vi "etlReadOpen.vi"   [LabVIEW 2017]
uses:
  globalDevices.vi
  <vilib>/DAQmx/create/channels.llb/DAQmx Create Channel (AI-Voltage-Basic).vi
  <vilib>/DAQmx/configure/timing.llb/DAQmx Timing (Sample Clock).vi
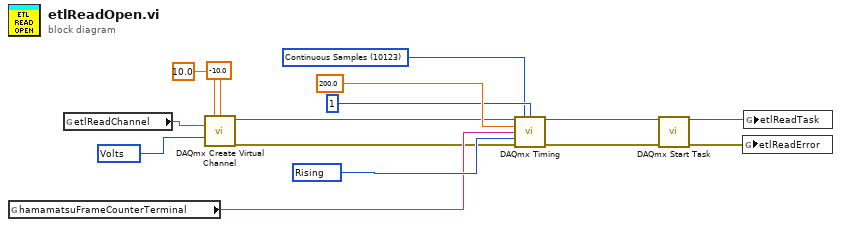
[diagram p0: block diagram]
diagram:
  w10 = 10348 items=["Volts"=10348, "From Custom Scale"=10065] ("units")
  w15 = 10280 items=["Rising"=10280, "Falling"=10171] ("active edge")
  w11 = 10123 items=["Finite Samples"=10178, "Continuous Samples"=10123, "Hardware Timed Single Point"=12522] ("sample mode")
  n1 = global read "globalDevices.vi" "hamamatsuFrameCounterTerminal"() -> (w14:tag)
  n2 = global read "globalDevices.vi" "etlReadChannel"() -> (w1:tag)
  n3 = call-poly <vilib>:"DAQmx Create Virtual Channel.vi"("maximum value"=10.0, "minimum value"=-10.0, "physical channels"=w1, "units"=w10) -> ("task out"=w6:refnum<k21>, "error out"=w7:errorcluster)  [unwired: 10 in]
  n4 = call-poly <vilib>:"DAQmx Timing.vi"("task/channels in"=w6, "sample mode"=w11, "samples per channel"=1, "rate"=200.0, "source"=w14, "active edge"=w15, "error in"=w7) -> ("task out"=w8:refnum<k21>, "error out"=w9:errorcluster)  [unwired: 7 in]
  n5 = call <vilib>:"DAQmx Start Task.vi"("task/channels in"=w8, "error in"=w9) -> ("task out"=w3:refnum<k21>, "error out"=w2:errorcluster)  [unwired: 12 in]
  n6 = global write "globalDevices.vi" "etlReadError"(w2) -> ()
  n7 = global write "globalDevices.vi" "etlReadTask"(w3) -> ()
